vi "Thev-Adjust Length.vi"(0 "history":cluster{dbl[], dbl[]}, 5 "Pos":dbl, 7 "Actual":dbl, 9 "Freq":dbl) -> (8 "Pos out":dbl)   [LabVIEW 2015]
uses:
  <vilib>/Analysis/NI_AALPro.lvlib
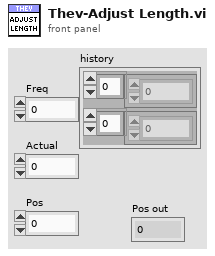
[diagram p1: front panel]
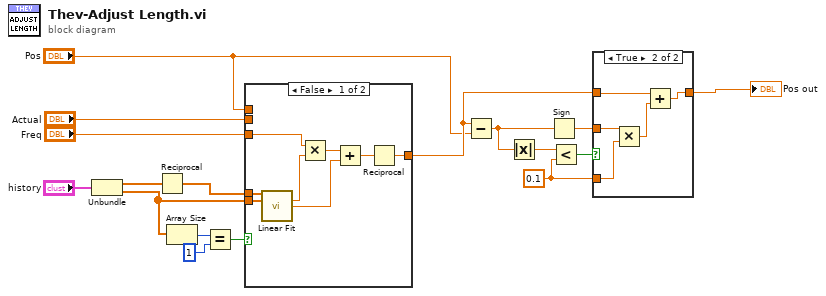
[diagram p0: block diagram]
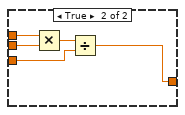
[diagram p2: hidden frame]
diagram:
  w13 = 0.1
  n1 = Unbundle("history") -> (w10:dbl[], w6:dbl[])
  n2 = Reciprocal(x=w10) -> (1/x=w9:dbl[])
  n3 = Array Size(array=w6) -> (size(s)=w5:i32)
  n4 = Equal?(x=w5, y=1) -> (x = y?=w3:bool)
  n5 = case shown="False" w3 {
    tunnel: w9 -> [w25 _]
    tunnel: "Freq" -> [w24 w27]
    tunnel: [w18 w26] -> w7
    tunnel: w6 -> [w19 _]
    tunnel: "Pos" -> [_ w30]
    tunnel: "Actual" -> [_ w29]
    frame False {
      n6 = call <vilib>:"Linear Fit.vi"("Y"=w25, "X"=w19) -> ("slope"=w23:dbl, "intercept"=w21:dbl)  [unwired: 9 in, 3 out]
      n7 = Multiply(x=w24, y=w23) -> (x*y=w22:dbl)
      n8 = Add(x=w22, y=w21) -> (x+y=w20:dbl)
      n9 = Reciprocal(x=w20) -> (1/x=w18:dbl)
    }
    frame True {
      n10 = Multiply(x=w30, y=w29) -> (x*y=w28:dbl)
      n11 = Divide(x=w28, y=w27) -> (x/y=w26:dbl)
    }
  }
  n12 = Subtract(x=w7, y="Pos") -> (x-y=w15:dbl)
  n13 = Absolute Value(x=w15) -> (abs(x)=w17:dbl)
  n14 = Sign(1:w15) -> (0:w14:dbl)
  n15 = Less?(x=w17, y=w13) -> (x < y?=w16:bool)
  n16 = case shown="True" w16 {
    tunnel: w7 -> [w31 w33]
    tunnel: w14 -> [_ w36]
    tunnel: w13 -> [_ w35]
    tunnel: [w31 w32] -> w12
    frame False {
    }
    frame True {
      n17 = Multiply(x=w36, y=w35) -> (x*y=w34:dbl)
      n18 = Add(x=w33, y=w34) -> (x+y=w32:dbl)
    }
  }
  "Pos out" <- w12
